vi "Refs_Initial.vi"(7 "Refs cluster In":T1) -> (3 "Refs cluster Out":T1)   [LabVIEW 2015]
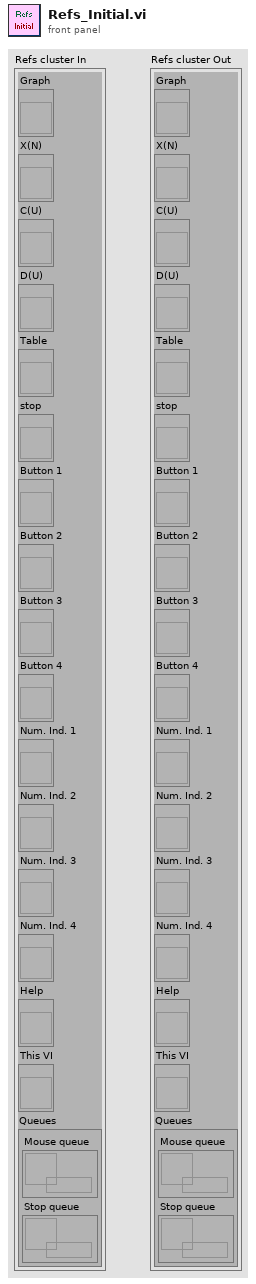
[diagram p1: front panel]
types:
  T1 = cluster{"Graph":refnum<vi>, "X(N)":refnum<vi>, "C(U)":refnum<vi>, "D(U)":refnum<vi>, "Table":refnum<vi>, "stop":refnum<vi>, "Button 1":refnum<vi>, "Button 2":refnum<vi>, "Button 3":refnum<vi>, "Button 4":refnum<vi>, "Num. Ind. 1":refnum<vi>, "Num. Ind. 2":refnum<vi>, "Num. Ind. 3":refnum<vi>, "Num. Ind. 4":refnum<vi>, "Help":refnum<vi>, "This VI":refnum<vi>, "Queues":cluster{"Mouse queue":refnum<queue>, "Stop queue":refnum<queue>}}
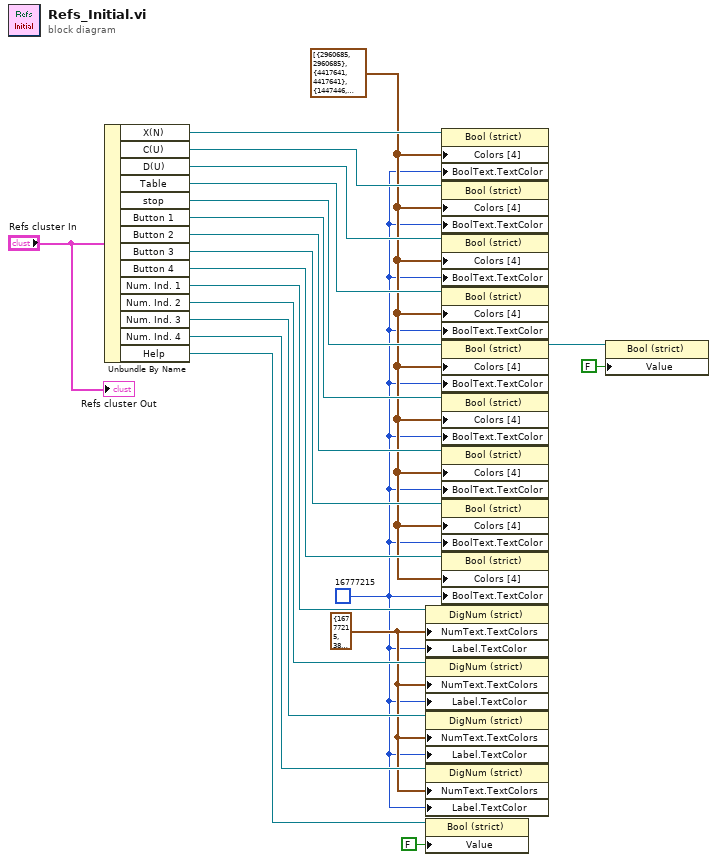
[diagram p0: block diagram]
diagram:
  w8 = cluster{u32, u32}[] [{2960685, 2960685}, {4417641, 4417641}, {1447446, 1447446}, {2176052, 2176052}] ("Not over colors")
  w6 = u32 16777215
  w7 = cluster{u32, u32} {16777215, 3815994} ("Cluster")
  n1 = Unbundle By Name("Refs cluster In") -> ("X(N)"=w21:refnum<vi>, "C(U)"=w20:refnum<vi>, "D(U)"=w19:refnum<vi>, "Table"=w18:refnum<vi>, "stop"=w17:refnum<vi>, "Button 1"=w16:refnum<vi>, "Button 2"=w15:refnum<vi>, "Button 3"=w14:refnum<vi>, "Button 4"=w13:refnum<vi>, "Num. Ind. 1"=w12:refnum<vi>, "Num. Ind. 2"=w11:refnum<vi>, "Num. Ind. 3"=w10:refnum<vi>, "Num. Ind. 4"=w9:refnum<vi>, "Help"=w4:refnum<vi>)
  n2 = property on="Property Node" class="DigNum (strict)"(reference=w12, "NumText.TextColors"=w7, "Label.TextColor"=w6) -> ()  [unwired: 1 in, 2 out]
  n3 = property on="Property Node" class="DigNum (strict)"(reference=w11, "NumText.TextColors"=w7, "Label.TextColor"=w6) -> ()  [unwired: 1 in, 2 out]
  n4 = property on="Property Node" class="DigNum (strict)"(reference=w10, "NumText.TextColors"=w7, "Label.TextColor"=w6) -> ()  [unwired: 1 in, 2 out]
  n5 = property on="Property Node" class="DigNum (strict)"(reference=w9, "NumText.TextColors"=w7, "Label.TextColor"=w6) -> ()  [unwired: 1 in, 2 out]
  n6 = property on="Property Node" class="Bool (strict)"(reference=w4, "Value"=FALSE) -> ()  [unwired: 1 in, 2 out]
  n7 = property on="Property Node" class="Bool (strict)"(reference=w21, "Colors [4]"=w8, "BoolText.TextColor"=w6) -> ()  [unwired: 1 in, 2 out]
  n8 = property on="Property Node" class="Bool (strict)"(reference=w20, "Colors [4]"=w8, "BoolText.TextColor"=w6) -> ()  [unwired: 1 in, 2 out]
  n9 = property on="Property Node" class="Bool (strict)"(reference=w19, "Colors [4]"=w8, "BoolText.TextColor"=w6) -> ()  [unwired: 1 in, 2 out]
  n10 = property on="Property Node" class="Bool (strict)"(reference=w18, "Colors [4]"=w8, "BoolText.TextColor"=w6) -> ()  [unwired: 1 in, 2 out]
  n11 = property on="Property Node" class="Bool (strict)"(reference=w17, "Colors [4]"=w8, "BoolText.TextColor"=w6) -> (reference out=w3:refnum<vi>)  [unwired: 1 in, 1 out]
  n12 = property on="Property Node" class="Bool (strict)"(reference=w16, "Colors [4]"=w8, "BoolText.TextColor"=w6) -> ()  [unwired: 1 in, 2 out]
  n13 = property on="Property Node" class="Bool (strict)"(reference=w15, "Colors [4]"=w8, "BoolText.TextColor"=w6) -> ()  [unwired: 1 in, 2 out]
  n14 = property on="Property Node" class="Bool (strict)"(reference=w14, "Colors [4]"=w8, "BoolText.TextColor"=w6) -> ()  [unwired: 1 in, 2 out]
  n15 = property on="Property Node" class="Bool (strict)"(reference=w13, "Colors [4]"=w8, "BoolText.TextColor"=w6) -> ()  [unwired: 1 in, 2 out]
  n16 = property on="Property Node" class="Bool (strict)"(reference=w3, "Value"=FALSE) -> ()  [unwired: 1 in, 2 out]
  "Refs cluster Out" <- "Refs cluster In"
